vi "sync.acknowledgement.vi"(8 "error in (no error)":errorcluster, 11 "synchronization":refnum<class "synchronization.lvclass">) -> (0 "error out":errorcluster, 3 "synchronization out":refnum<class "synchronization.lvclass">)   [LabVIEW 2020, in "synchronization.lvclass"]
uses:
  synchronization.lvclass
  synchronization.lvclass/synchronization.ctl
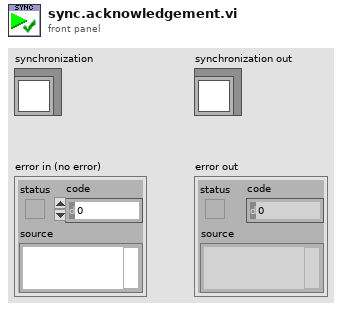
[diagram p1: front panel]
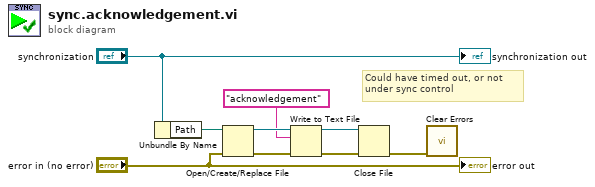
[diagram p0: block diagram]
diagram:
  # "Could have timed out, or not under sync control"
  n1 = Unbundle By Name("synchronization") -> ("Path"=w4:path)
  n2 = Open/Create/Replace File(file path (use dialog)=w4, error in="error in (no error)") -> (refnum out=w8:refnum<file>, error out=w7:errorcluster)  [unwired: 4 in, 1 out]
  n3 = Write to Text File(file (use dialog)=w8, text="acknowledgement", error in=w7) -> (refnum out=w6:refnum<file>, error out=w5:errorcluster)  [unwired: 1 in, 1 out]
  n4 = Close File(refnum=w6, error in=w5) -> (error out=w3:errorcluster)  [unwired: 1 out]
  n5 = call <vilib>:"Clear Errors.vi"("error in (no error)"=w3) -> ()  [unwired: 5 in, 2 out]
  "error out" <- "error in (no error)"
  "synchronization out" <- "synchronization"
